vi "2-2.vi"() -> ()   [LabVIEW 2019, in "AoC2022.lvlib"]
uses:
  AoC2022.lvlib
panel:
  out "Player 1":i32
  out "Player 2":i32
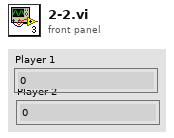
[diagram p1: front panel]
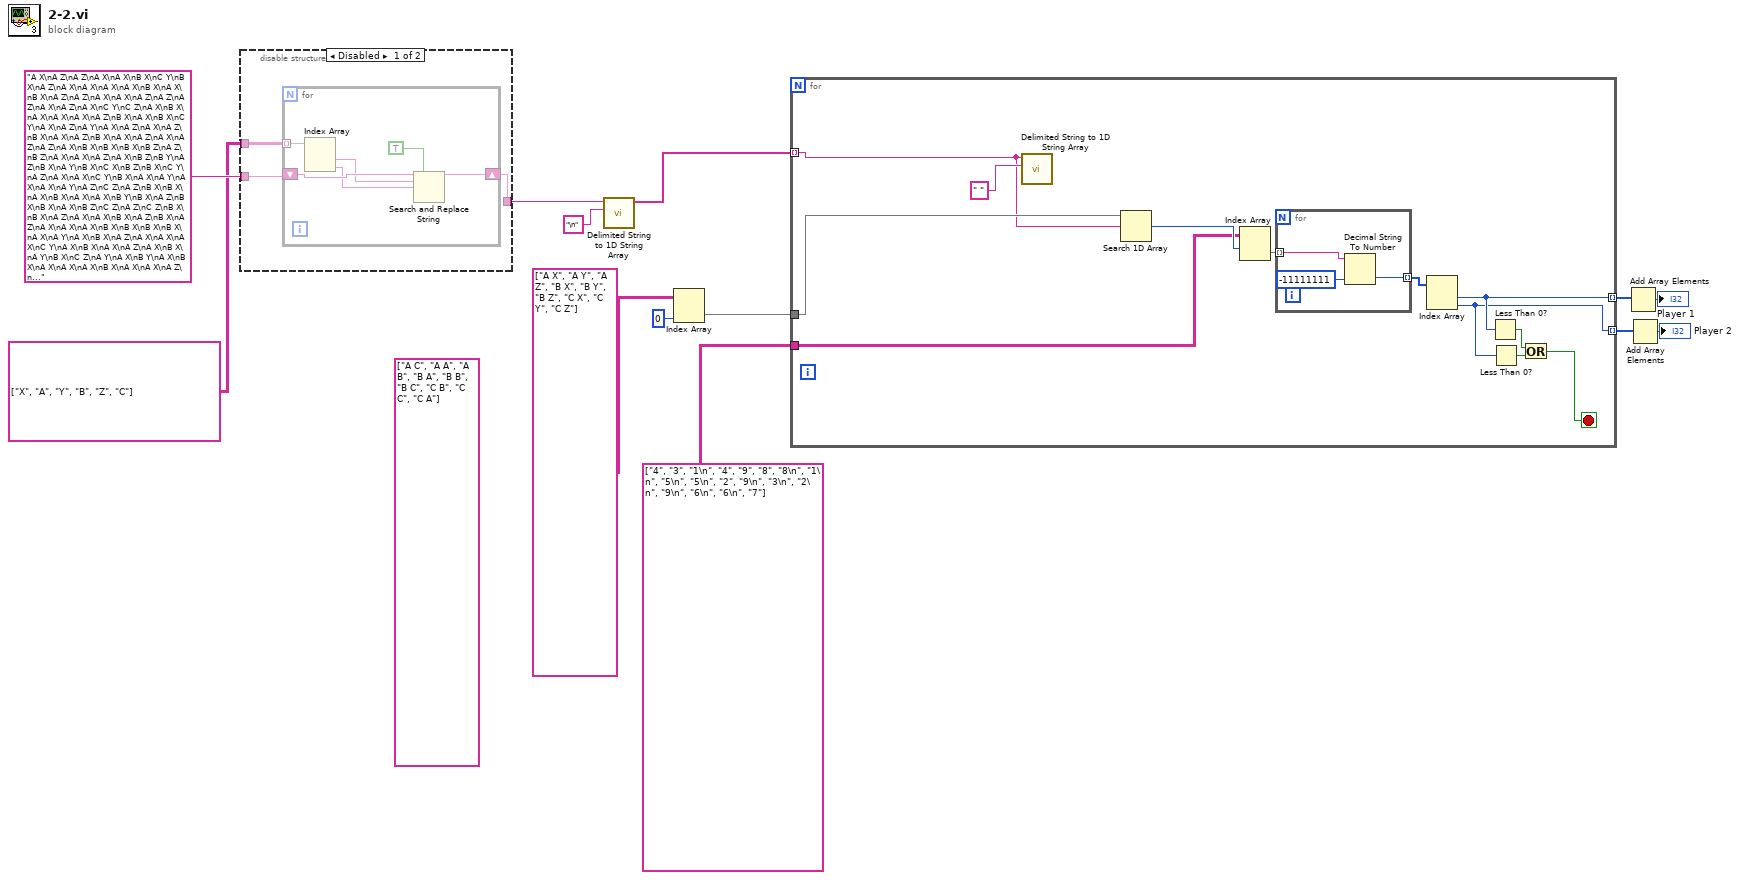
[diagram p0: block diagram]
diagram:
  (unwired) string[][] [["A C"], ["A A"], ["A B"], ["B A"], ["B B"], ["B C"], ["C B"], ["C C"], ["C A"]]
  n1 = disable-structure shown="Disabled" {
    disable-tunnel: "A X\nA Z\nA Z\nA X\nA X\nB X\nC Y\nB X\nA Z\nA X\nA X\nA X\nA X\nB X\nA X\nB X\nA Z\nA Z\nA X\nA X\nA Z\nA Z\nA Z\nA X\nA Z\nA X\nC Y\nC Z\nA X\nB X\nA X\nA X\nA X\nA Z\nB X\nA X\nB X\nC Y\nA X\nA Z\nA Y\nA X\nA Z\nA X\nA Z\nB X\nA X\nA Z\nB X\nA X\nA Z\nA X\nA Z\nA Z\nA X\nB X\nB X\nB X\nB Z\nA Z\nB Z\nA X\nA X\nA Z\nA X\nB Z\nB Y\nA Z\nB X\nA Y\nB X\nC X\nB Z\nB X\nC Y\nA Z\nA X\nA X\nC Y\nB X\nA X\nA Y\nA X\nA X\nA Y\nA Z\nC Z\nA Z\nB X\nB X\nA X\nB X\nA X\nA X\nB Y\nB X\nA Z\nB X\nB X\nA X\nB Z\nC Z\nA Z\nC Z\nB X\nB X\nA Z\nA X\nA X\nB X\nA Z\nB X\nA Z\nA X\nA X\nA X\nB X\nB X\nB X\nB X\nA X\nA Y\nA X\nB X\nA Z\nA X\nA X\nA X\nC Y\nA X\nB X\nA X\nA Z\nA X\nB X\nA Y\nB X\nC Z\nA Y\nA X\nB Y\nA X\nB X\nA X\nA X\nA X\nB X\nA X\nA X\nA Z\nA Z\nA X\nC Y\nB X\nB X\nA Z\nB X\nB Y\nC Y\nA X\nA X\nB Y\nA X\nB Y\nB X\nB X\nA X\nA Z\nB X\nB X\nA Y\nA X\nC Y\nC Y\nC Y\nA X\nB X\nA X\nA X\nA X\nB X\nB X\nC Y\nA X\nA Z\nA Z\nA X\nB X\nA Z\nA Z\nA X\nB X\nA X\nA Z\nA X\nC Z\nB X\nA X\nC Y\nC Y\nA Z\nB X\nB Z\nC Y\nB X\nA Y\nB Y\nA Z\nA X\nA X\nB X\nB Y\nA Z\nA X\nB X\nA X\nC X\nC Y\nA X\nB X\nA Z\nA X\nB X\nA X\nC Y\nC Y\nC Y\nA X\nA X\nA Z\nA X\nC Y\nA Z\nB Y\nA X\nC Y\nB Z\nB X\nB X\nA Z\nB X\nA Y\nC X\nA X\nB X\nA Z\nC Y\nA X\nA Z\nC Z\nA X\nC Y\nB X\nC Y\nC Z\nA Y\nA Z\nC Y\nA X\nA X\nA X\nA Y\nB X\nB X\nC Y\nC Y\nA X\nA Z\nC Y\nB Z\nB X\nC Z\nB X\nB X\nC Z\nA X\nA X\nB X\nB X\nA X\nA X\nB X\nB X\nB X\nC Y\nA X\nA X\nA X\nA X\nB X\nA X\nA X\nB X\nB Z\nA X\nB X\nA X\nC Y\nB Y\nA X\nB X\nA Y\nB Z\nB X\nA X\nB Z\nB X\nA Y\nA X\nB X\nA X\nA Z\nB X\nA X\nA X\nC Z\nA X\nB X\nA X\nB Y\nA Z\nA X\nB X\nA X\nA Z\nB X\nB X\nB Y\nB X\nA X\nC Y\nA X\nA X\nB X\nB Y\nA X\nA X\nA X\nC Z\nC Z\nB Y\nB X\nB Z\nA X\nA Y\nA X\nC Y\nB X\nA X\nA X\nA X\nA Z\nC Y\nA X\nA X\nC Y\nA X\nA X\nA X\nA Z\nA Y\nA X\nA Y\nC Z\nA Z\nA X\nB X\nA Z\nC Z\nC Y\nA Z\nA Z\nC Y\nC Z\nC Z\nA X\nB X\nB X\nB Z\nC Y\nA X\nA X\nA X\nA Z\nA X\nB X\nB X\nC X\nA X\nA X\nB X\nA Y\nA X\nA X\nB Y\nC Z\nA X\nA X\nA Y\nB X\nB X\nB X\nC Z\nA Z\nA Y\nB Y\nA X\nB X\nB X\nB X\nB Z\nA Y\nB Y\nA Z\nA Z\nC Z\nB X\nA X\nA Y\nA Y\nC Y\nB Y\nA X\nA X\nA X\nA X\nB Y\nA X\nA Y\nA X\nA Z\nB X\nB X\nA Y\nA X\nA Y\nA Y\nA Z\nB X\nB X\nA Z\nB X\nA X\nA Z\nA Z\nB X\nA Z\nA X\nA Y\nA Z\nA X\nA Z\nB Y\nA X\nC Y\nB X\nC X\nC Y\nB Z\nC Y\nC Y\nA X\nA X\nA Y\nB X\nC Z\nB X\nC Y\nA X\nA Z\nC Y\nA X\nA Z\nA Z\nB Y\nA X\nA X\nB X\nB Y\nA X\nA X\nB X\nA X\nB X\nA X\nB X\nA X\nB Y\nA Z\nB X\nB X\nB X\nB X\nA Y\nA X\nA Y\nA Y\nC Z\nB Z\nA X\nB Y\nA X\nC Z\nB X\nA X\nA X\nA X\nA X\nA X\nC Z\nC Z\nC Z\nA X\nC Y\nA X\nC X\nC Z\nA X\nB X\nA Z\nA Z\nA Z\nA X\nA Z\nA Z\nB Z\nA X\nB X\nA Z\nC Y\nA X\nA Z\nA Z\nA Z\nB Z\nB X\nA X\nB X\nB X\nB X\nB X\nB Y\nB X\nA X\nA X\nA Z\nA Z\nA Z\nB Y\nA X\nA X\nA Y\nB X\nB X\nA Z\nA X\nB X\nA X\nA X\nA Z\nC Y\nA X\nB X\nA X\nB X\nA X\nB X\nA Z\nB X\nA X\nA Z\nA Z\nB X\nA Y\nA X\nA Z\nC Y\nA X\nA X\nA X\nB Y\nB X\nA Y\nA Z\nC X\nB X\nC Y\nA X\nB X\nC Z\nC Z\nA X\nB X\nB X\nB Y\nB X\nB X\nA X\nA Z\nB Z\nB X\nA X\nB X\nB X\nB X\nA Z\nA X\nA X\nA Z\nB Y\nB Z\nA X\nA Z\nA Z\nA Z\nA X\nA X\nA X\nA X\nA X\nA X\nB X\nA Z\nB Z\nA X\nA Z\nC Y\nA Z\nA X\nA Y\nA Y\nB X\nB Y\nA Z\nA X\nB X\nB Y\nA X\nB X\nA X\nB X\nB X\nC Y\nA Z\nB X\nA X\nB X\nA X\nA Z\nA X\nA Z\nA X\nA X\nA X\nB X\nA Y\nA X\nA X\nB X\nC Z\nB X\nA X\nC Y\nA X\nB X\nA Z\nB Y\nB Z\nA X\nA X\nA X\nC Y\nA X\nA X\nA X\nB X\nC Z\nA Z\nA X\nC Z\nB X\nA Z\nA Y\nC Y\nC Y\nA Z\nB X\nC Z\nC Z\nA X\nA X\nA X\nA X\nA X\nB X\nC Y\nA Z\nA X\nB X\nA Z\nA X\nA Y\nA X\nB Z\nA X\nB X\nA X\nA X\nA X\nA Y\nB X\nC Y\nA X\nA Z\nC Y\nA Z\nA X\nA Y\nA X\nA Z\nA X\nA Y\nC Y\nA Y\nA Z\nA X\nA X\nA X\nA Z\nA X\nB X\nA Y\nA X\nB X\nA X\nA X\nB X\nA X\nB X\nC Z\nB X\nA Z\nA Z\nC Y\nB Y\nB X\nA Y\nB X\nB X\nA Y\nA X\nC X\nC Y\nB X\nA X\nC X\nC Z\nA X\nA Z\nB X\nB Z\nC Y\nA X\nC Y\nA Y\nB X\nB Y\nA X\nC Y\nA Z\nA X\nA X\nC Y\nC Y\nA X\nA Z\nB X\nA Y\nB X\nA Z\nA Z\nA Z\nA Z\nA X\nC Z\nB X\nB Y\nA X\nA Y\nA X\nB X\nC Y\nC Z\nB Z\nB X\nB Z\nA X\nA Z\nC Y\nA X\nB Y\nA X\nA Z\nA X\nC Z\nA X\nA Y\nB Y\nA X\nA X\nA X\nA Z\nB X\nB X\nB X\nA X\nC Y\nC X\nC Y\nC Z\nA X\nA X\nA Z\nA Z\nA X\nA X\nA X\nA X\nA X\nA X\nA X\nC Z\nA X\nB X\nA Z\nB X\nB X\nB X\nA Y\nA X\nA X\nB X\nA X\nB X\nA Z\nC Y\nB Y\nC Z\nB Y\nB X\nB X\nA X\nC Z\nA X\nB Y\nC Y\nB Y\nA Z\nA Y\nA X\nA X\nC Y\nB X\nB X\nA Z\nA X\nC Y\nC Y\nA Y\nA Z\nB X\nC Z\nA Z\nC Y\nA X\nA X\nA Z\nB X\nA X\nA X\nA Z\nB X\nC Z\nA X\nA X\nB X\nB Y\nA Z\nA X\nB X\nA X\nC Y\nB X\nB X\nB Z\nC Y\nA X\nB X\nA X\nA X\nA Y\nA Y\nA Z\nB X\nA Z\nB Y\nB X\nA X\nB Y\nA X\nA X\nA Z\nA X\nB X\nA Z\nA X\nA Z\nB X\nB X\nB X\nB Z\nC Y\nA Y\nA Y\nA Z\nA X\nB X\nB X\nA X\nA X\nB Y\nA X\nB X\nA Z\nB Z\nB X\nC Y\nA Z\nA X\nC Z\nA Y\nA Y\nB X\nA Y\nC Z\nA Z\nA X\nB X\nA Z\nC Y\nC X\nB X\nB Z\nA X\nA Y\nA X\nB X\nA X\nA X\nC Y\nB Z\nB Z\nB Y\nC Z\nC Y\nB X\nB Y\nC Y\nA Z\nB X\nA X\nA X\nA X\nA X\nA X\nA X\nB X\nB X\nB X\nA X\nC Y\nA X\nA Y\nA Z\nB Y\nC Y\nA Z\nA X\nA X\nA Z\nA Y\nB X\nA Y\nA X\nA X\nC Z\nA X\nA X\nB X\nA X\nA Z\nA Z\nA X\nA X\nA X\nB X\nA X\nA X\nA X\nA Z\nA X\nB X\nB Z\nC Y\nA X\nA Z\nB X\nB X\nB X\nA X\nB X\nA X\nB X\nA Y\nB Y\nC Y\nA X\nC Z\nB Z\nA Z\nA X\nA X\nA Z\nA Y\nA Z\nA X\nA X\nB X\nA X\nA X\nA Z\nC Z\nB X\nB Y\nA Z\nB X\nA Z\nA X\nA X\nA X\nC Y\nC Y\nA Z\nA X\nA X\nB Y\nA Y\nA X\nB Z\nB X\nB Z\nB X\nB Y\nB X\nA Y\nA Z\nC Y\nB X\nA X\nA X\nB X\nB Z\nA X\nC X\nA X\nA X\nA X\nA X\nA X\nA X\nB X\nA X\nC Z\nA Y\nB X\nB X\nB Z\nA X\nB X\nB Z\nB X\nA Z\nA X\nB X\nA X\nA Y\nB X\nA Z\nC Z\nB X\nC Z\nA X\nA X\nC Y\nA Z\nC Y\nA Z\nA X\nB X\nA X\nC Y\nA Z\nA X\nA X\nB X\nB X\nA Z\nB Y\nB X\nA X\nA Z\nA X\nB X\nA X\nA Z\nA Z\nA Y\nA Y\nA X\nC Z\nA Z\nA Z\nA X\nB X\nA Y\nB Z\nA X\nA Z\nA X\nC Z\nB X\nA Z\nC Z\nA X\nC X\nA Z\nA X\nA X\nB Z\nA X\nB X\nA X\nB X\nC Z\nA X\nB X\nA Z\nB X\nC Y\nB X\nA Z\nA X\nA Y\nC Z\nA Z\nB X\nA Z\nA Y\nA Z\nB X\nA X\nB X\nC Y\nB X\nA X\nC Y\nA X\nA X\nB Y\nA X\nB Y\nA X\nA X\nA X\nB X\nA X\nA X\nC Z\nA X\nB X\nA Y\nA Y\nB Z\nA Z\nA Y\nA X\nB X\nB Y\nA Z\nB Y\nA X\nA Z\nA X\nA Z\nB X\nA X\nA X\nB X\nA Y\nB X\nB X\nA X\nA Z\nB X\nA Y\nB X\nA Z\nB X\nB X\nB X\nB X\nA Y\nA Z\nB X\nB Y\nB X\nC Y\nC Y\nC Y\nB X\nB X\nA Y\nA X\nB X\nB X\nA X\nB X\nA X\nA Z\nA Z\nA Z\nB X\nA X\nA X\nA Y\nA X\nA X\nC Y\nB X\nC Y\nA X\nA Y\nC Z\nA X\nB X\nA Z\nA X\nA X\nA Z\nA X\nB Z\nA X\nA Z\nA X\nC Y\nA Y\nC X\nA X\nC Y\nB X\nB X\nA Z\nA X\nA X\nA X\nB X\nA X\nC Y\nC Y\nA Y\nA X\nC Z\nA X\nB X\nB Y\nA Z\nA X\nB X\nB X\nA X\nA Z\nC Y\nB X\nA Y\nA X\nA Z\nB X\nA X\nA Z\nB X\nA Y\nB Z\nA Z\nC Z\nC Y\nA Z\nA X\nA X\nA Z\nB X\nA X\nB X\nA X\nA X\nB X\nA Z\nA X\nC Z\nB X\nA Z\nB Y\nA Z\nA X\nA Z\nB X\nA X\nA X\nA Y\nB X\nC Z\nB X\nA X\nA X\nA Z\nB X\nC X\nB X\nB X\nA Z\nB Y\nB X\nA Z\nC Y\nA X\nA X\nB X\nB X\nA X\nB X\nA Z\nA X\nA X\nA Z\nA X\nA X\nB X\nB X\nA X\nA Z\nA Y\nA X\nA X\nC Y\nB X\nA X\nB X\nC Z\nA Z\nB X\nA X\nA X\nA X\nC Y\nA X\nA X\nA X\nA Z\nB Y\nB X\nA X\nA X\nA Z\nB X\nC Z\nB X\nA Z\nA Z\nA X\nA Y\nB Y\nB X\nA Z\nA Z\nA X\nA Y\nB X\nA X\nA Z\nB X\nA Y\nA Z\nA Z\nB X\nC Z\nA X\nA X\nB X\nB X\nA X\nA Y\nA Y\nC Z\nB X\nA X\nA Z\nC Y\nB X\nA Z\nA X\nB X\nB Y\nA X\nB X\nA Y\nB X\nA X\nA Z\nB X\nB X\nC Y\nB X\nB X\nB Y\nA X\nA X\nB X\nB X\nA X\nB X\nC Y\nA X\nA X\nA Z\nA Z\nB X\nA Y\nB X\nB Y\nA X\nA Z\nA X\nA Z\nA X\nB Y\nB X\nB X\nA X\nB X\nA X\nB X\nB X\nA X\nB X\nC X\nA Z\nA Z\nA X\nA X\nA Z\nA X\nB X\nA X\nA X\nA Z\nA Z\nA X\nA X\nB X\nC Y\nA Z\nA X\nA X\nA Y\nA X\nB Z\nC Z\nA Z\nB X\nA X\nB X\nA X\nB X\nB X\nA Y\nB Y\nA X\nB X\nB Y\nC Y\nB Z\nB Y\nB Y\nA Z\nA X\nA Y\nA X\nA Z\nA Z\nA X\nA X\nA X\nA X\nA Y\nC Y\nA X\nA Y\nA Z\nA Z\nB X\nA X\nA X\nA Z\nB Y\nB X\nB X\nA X\nB Z\nB Z\nA Y\nB X\nA Y\nA X\nB X\nC Z\nA X\nA Y\nB X\nA X\nB Z\nC Y\nA Z\nA X\nA Z\nA X\nA X\nA X\nA X\nC Y\nB X\nA X\nA X\nC Y\nC Y\nA Z\nC Y\nA Z\nA Y\nC X\nB X\nC Y\nA Z\nA X\nB X\nB Z\nB X\nB X\nB X\nB X\nB X\nA X\nA Z\nB X\nA Y\nA X\nA Y\nB X\nA X\nA X\nA X\nB Z\nB Z\nB X\nB X\nA Y\nA X\nB Y\nB X\nB Y\nC Y\nA X\nA X\nC Y\nA X\nB X\nB X\nB X\nC Z\nB X\nA Z\nB X\nB X\nA X\nB Z\nA Z\nA Z\nA X\nA Z\nA Y\nA Z\nB X\nA X\nB X\nA X\nA X\nA X\nB X\nA X\nB X\nA X\nA X\nB X\nA Z\nA X\nA Z\nC Y\nA X\nB X\nA X\nA X\nB X\nB X\nC Z\nA X\nA X\nB X\nA X\nA Y\nA X\nA X\nA Z\nA X\nA X\nB X\nA X\nA X\nA X\nA Y\nC Z\nA Z\nA Z\nA X\nB X\nA Z\nA X\nA X\nA X\nC Y\nC Y\nA Z\nC Y\nB X\nA X\nB X\nB X\nA Z\nA Z\nA Y\nB X\nA Z\nA X\nA Z\nA X\nA X\nA X\nA Z\nA Z\nB X\nA X\nA X\nB X\nB X\nA Z\nB X\nA X\nA X\nB X\nB X\nB X\nA X\nA X\nA Z\nA X\nA X\nB Y\nB Y\nC Y\nA Y\nA Y\nB X\nB X\nC Y\nA X\nB X\nA X\nA X\nA Z\nA Y\nA X\nB X\nA X\nB X\nA X\nA Z\nA X\nC Y\nB X\nB X\nA X\nB X\nA X\nA X\nA Z\nC Y\nB X\nB X\nA X\nA X\nA Z\nA Z\nB Y\nA X\nB X\nA Y\nC Z\nB X\nA X\nA Z\nB Y\nA Z\nB X\nB X\nB X\nA X\nA Z\nA Z\nB Y\nA Y\nB X\nB Y\nA Y\nA Z\nA X\nA X\nB X\nB X\nA Y\nB X\nA X\nA X\nC Y\nB X\nA X\nC X\nC Z\nA X\nA X\nC Y\nC Z\nA Z\nA X\nC Y\nC Y\nC Y\nA X\nA Y\nA Z\nA X\nC Z\nA X\nC X\nB X\nB Y\nB Z\nA X\nA X\nA X\nA Z\nB X\nB X\nC X\nA X\nC Z\nC Y\nA X\nA X\nB X\nB X\nA X\nA X\nA X\nA Z\nA Z\nB X\nA Z\nB Y\nA Y\nA Y\nA Z\nB X\nA Y\nA X\nA X\nB X\nA Z\nB X\nA Y\nA X\nB X\nA X\nB X\nA X\nB X\nB Z\nA Z\nA Y\nA Z\nA X\nB X\nB X\nC Y\nB X\nA X\nB X\nA Y\nB X\nB X\nC Y\nB X\nA Z\nA Z\nC Y\nA X\nB X\nB X\nA X\nB X\nA Z\nA X\nA X\nA Z\nA Z\nC Z\nA X\nA X\nA X\nA X\nA X\nA X\nA Z\nC Y\nA X\nC Y\nA X\nB X\nC Y\nB X\nA Y\nB X\nB X\nB X\nA X\nA X\nA X\nC Y\nA Z\nA Z\nB X\nA X\nA Z\nB X\nB X\nA X\nA X\nB Z\nA X\nB Z\nB X\nA X\nA X\nA X\nB X\nA X\nC Y\nA Y\nA X\nA X\nB X\nA Y\nA X\nC Y\nC Y\nB X\nB X\nA X\nA X\nC Y\nB Y\nC Y\nA X\nB X\nA Y\nB Z\nB X\nB X\nA Y\nB X\nA Z\nC Y\nB X\nB X\nB Y\nA X\nA X\nA X\nC Y\nB X\nA Y\nB X\nA Z\nB Y\nA X\nA X\nA X\nA X\nA X\nA X\nB X\nC Z\nB X\nB X\nA X\nA X\nC Y\nA X\nA X\nA X\nA X\nB Z\nB X\nA Z\nB Z\nC Z\nC Y\nB X\nB X\nC Z\nA Z\nA Y\nA Z\nA Y\nC Z\nA X\nA X\nA Z\nA X\nA Z\nA X\nB Z\nB X\nB X\nC Z\nB X\nC Y\nC Y\nB X\nA X\nA X\nA X\nB Y\nA X\nC Y\nB Y\nC Y\nB Y\nA Z\nB X\nA X\nA Z\nB X\nB Z\nA Z\nA X\nA X\nA Y\nA X\nA X\nA Z\nB X\nB X\nB X\nB X\nB X\nA X\nA X\nA X\nA Z\nA Z\nA Y\nA X\nA Z\nA Z\nB X\nA X\nB X\nB X\nA Z\nB Y\nA X\nA X\nA X\nA X\nB X\nA Y\nA X\nC X\nA Z\nA X\nC Z\nC Y\nB X\nA Z\nA Z\nB X\nC Y\nA X\nA Z\nA X\nB Y\nC Y\nA X\nA X\nA Z\nA X\nC Y\nA Z\nA X\nA X\nA X\nC Y\nB X\nA X\nB Y\nA Z\nA X\nA Z\nB X\nA Z\nA Z\nA X\nA X\nC Z\nB X\nA Z\nA X\nB Z\nA Z\nA Z\nB X\nA X\nA Z\nA Y\nA X\nA Z\nA Z\nC X\nC Z\nB X\nB X\nA Z\nA X\nB X\nA X\nA X\nA X\nA Z\nB X\nA Z\nA X\nB X\nA X\nA X\nC Z\nB X\nC Y\nA X\nB X\nA Z\nA Z\nA X\nB Z\nB X\nA Z\nA Z\nA X\nC Y\nA X\nB X\nC Y\nB X\nB X\nA Z\nB X\nA Z\nC Y\nB X\nA Y\nB X\nA Z\nB Z\nA Z\nB X\nA X\nB Z\nA X\nA Y\nB Z\nC Y\nC Y\nB X\nA X\nA X\nA X\nA X\nB Z\nA X\nA X\nA X\nC Y\nC X\nB Y\nB X\nB X\nB X\nA Y\nA X\nA Z\nA X\nB X\nA Z\nC Y\nA X\nA Z\nA Z\nA X\nA X\nA X\nA X\nA Z\nA X\nA X\nB X\nC Z\nB X\nC Z\nB Y\nB X\nA Z\nA Z\nA Z\nB Y\nA Y\nA Z\nB X\nC Y\nA X\nB X\nA Z\nC Y\nA Y\nB X\nA X\nA Y\nA X\nA Z\nB X\nA Z\nB Y\nB X\nA X\nB X\nA X\nA X\nA X\nA Y\nB X\nA Y\nA X\nB X\nA X\nA X\nC Y\nA X\nA X\nB Z\nA Z\nA Z\nA X\nC Y\nB X\nB X\nC Y\nA Z\nC Y\nA X\nA X\nB X\nB X\nA X\nA Z\nB Y\nB X\nA Z\nB X\nA X\nB X\nA Z\nC Y\nA X\nB X\nA X\nA X\nA Z\nA X\nB X\nC Z\nA X\nA X\nA Y\nB X\nA Z\nB X\nB X\nB Y\nA X\nA Z\nA X\nA Z\nB X\nB X\nA X\nA X\nB Z\nA X\nC Y\nB X\nA X\nA Z\nA Z\nB X\nC Y\nC Y\nB Y\nA Z\nC Z\nA X\nB X\nA X\nA X\nB Y\nB X\nA X\nA X\nA Y\nA Z\nB X\nA X\nA X\nA Z\nA X\nA X\nB X\nB X\nA Y\nA X\nB X\nA Z\nB Z\nB X\nA Z\nA X\nA Z\nB X\nC Y\nA X\nA X\nB X\nA Z\nB X\nA Z\nC Z\nA Z\nA X\nC Y\nA X\nB X\nB Z\nA X\nB X\nC X\nA X\nB Y\nA X\nA X\nC Y\nA X\nB Y\nA X\nA X\nA X\nB X\nA X\nB X\nA Z\nC Y\nA X\nC Z\nA X\nB X\nA Z\nA X\nC Z\nC Z\nA X\nA Y\nA Z\nA X\nB X\nB X\nA Z\nB X\nA X\nB X\nB Y\nB X\nB X\nC Z\nA Y\nA X\nA Z\nB Z\nA X\nA Z\nA Z\nA Y\nB X\nA Y\nA X\nA X\nB X\nA Z\nB Z\nA X\nA Z\nA Z\nA Z\nC Y\nA X\nB Z\nB X\nA Z\nB X\nA Z\nA Y\nA X\nC Z\nC X\nA Y\nA X\nA Z\nA X\nA X\nA Z\nA Y\nA Z\nA Y\nA X\nC Y\nB X\nA Z\nA X\nA X\nC Y\nA X\nA X\nB Z\nA Z\nC Y\nA X\nA X\nA X\nB X\nC Y\nA X\nA Y\nB X\nA X\nA X\nB Y\nA Z\nA X\nA X\nB X\nA Z\nA Y\nC Y\nC Z\nC Y\nA X\nC Y\nC Y\nA X\nA Y\nC Y\nB X\nA X\nB X\nA X\nA X\nB X\nA X\nA Z\nC Y\nC Y\nB X\nA X\nB X\nC Z\nC Y\nB X\nA X\nA X\nA Y\nA X\nA Y\nA Z\nB X\nA Z\nA Z\nA X\nA X\nB X\nC Y\nB X\nA Z\nA X\nA X\nA X\nB X\nB Z\nB X\nB X\nB X\nA Z\nA X\nB Z\nA X\nB Z\nA X\nB Y\nC Z\nB Y\nC Z\nB Y\nB X\nA X\nA X\nC Y\nB X\nB X\nA X\nB Z\nA Z\nA Z\nA X\nA X\nA X\nB X\nB X\nB X\nC Y\nA X\nB X\nB X\nB Z\nB X\nA Z\nC Y\nA X\nC Z\nA Z" -> [w16 w23]
    disable-tunnel: string[][] [["X", "A"], ["Y", "B"], ["Z", "C"]] -> [w15 _]
    disable-tunnel: [w14 w23] -> w1
    frame Disabled {
      n2 = for {
        tunnel: w15 -> [w21] mode=indexing
        shift-right: [w17] -> w14
        shift-left: w16 -> [w22]
        n3 = Index Array(array=w21) -> (element #1=w20:string, element #2=w19:string)  [unwired: 2 in]
        n4 = Search and Replace String(replace all?=TRUE ("replace all? (F)"), input string=w22, search string=w20, replace string=w19) -> (result string=w17:string)  [unwired: 4 in, 3 out]
      }
    }
    frame Enabled {
    }
  }
  n5 = call <vilib>:"Delimited String to 1D String Array.vi"("delimiter"="\n", "delimited string"=w1) -> ("string array"=w12:string[])  [unwired: 9 in]
  n6 = Index Array(array=string[][] [["A X"], ["A Y"], ["A Z"], ["B X"], ["B Y"], ["B Z"], ["C X"], ["C Y"], ["C Z"]], index (col)=0 ("disabled index (col)")) -> (element=w9:string[])  [unwired: 1 in]
  n7 = for {
    tunnel: w12 -> [w33] mode=indexing
    tunnel: w9 -> [w34]
    tunnel: [w27] -> w8 mode=indexing
    tunnel: string[][] [["4", "3"], ["1\n", "4"], ["9", "8"], ["8\n", "1\n"], ["5\n", "5\n"], ["2", "9\n"], ["3\n", "2\n"], ["9\n", "6\n"], ["6\n", "7"]] -> [w31]
    tunnel: [w28] -> w4 mode=indexing
    stop <- w24 stop-if-true
    n8 = call <vilib>:"Delimited String to 1D String Array.vi"("delimiter"=" ", "delimited string"=w33) -> ()  [unwired: 9 in, 1 out]
    n9 = Search 1D Array(1D array=w34, element=w33) -> (index of element=w32:i32)  [unwired: 1 in]
    n10 = Index Array(array=w31, index (row)=w32) -> (element=w30:string[])  [unwired: 1 in]
    n11 = for {
      tunnel: [w38] -> w29 mode=indexing
      tunnel: w30 -> [w36] mode=indexing
      n12 = Decimal String To Number(string=w36, default (0L)=-11111111 ("default (0 I32)")) -> (number=w38:i32)  [unwired: 1 in, 1 out]
    }
    n13 = Index Array(array=w29) -> (element #1=w28:i32, element #2=w27:i32)  [unwired: 2 in]
    n14 = Less Than 0?(x=w28) -> (x < 0?=w25:bool)
    n15 = Less Than 0?(x=w27) -> (x < 0?=w26:bool)
    n16 = Or(x=w25, y=w26) -> (x .or. y?=w24:bool)
  }
  n17 = Add Array Elements(numeric array=w4) -> (sum=→"Player 1":i32)
  n18 = Add Array Elements(numeric array=w8) -> (sum=→"Player 2":i32)
